vi "Sweep Mode (Read).vi"(6 "ISOBUS address":T5=-1 caption="ISOBUS address (-1)", 8 "error in":errorcluster, 11 "Mercury Reference In":T2) -> (0 "error out":errorcluster, 2 "Sweep Mode":string, 3 "Mercury Reference Out":T2, 4 "Valid?":T1)   [LabVIEW 2013, in "Mercury iXX.lvlib" / "Control Loop.lvlib"]
doc: "Check the sweep mode of the control loop."
uses:
  <instrlib>/Mercury iXX/Public/Libraries/Control Loop.lvlib
  <instrlib>/Mercury iXX/Public/Controls/Mercury Reference.ctl
  <instrlib>/Mercury iXX/Public/Controls/Comms Transport Layer.ctl
  <instrlib>/Mercury iXX/Private/Controls/Query Dynamic Reference.ctl
  <instrlib>/Mercury iXX/Public/Controls/ISOBus Address.ctl
  <instrlib>/Mercury iXX/Public/Controls/Is Valid LED.ctl
  <instrlib>/Mercury iXX/Private/Controls/Command Verbs.ctl
  <instrlib>/Mercury iXX/Mercury iXX.lvlib
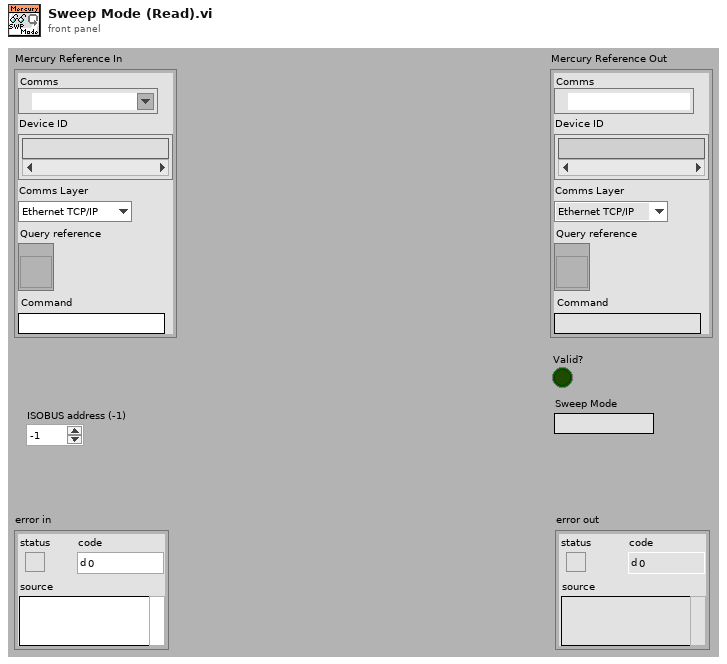
[diagram p1: front panel]
types:
  T1 = typedef "Mercury iXX.lvlib/Is Valid LED.ctl" = bool
  T2 = typedef "Mercury iXX.lvlib/Mercury Reference.ctl" = cluster{"Comms":refnum<visa-resource-name>, "Device ID":string[], "Comms Layer":T3, "Command":string, "Query reference":T4}
  T3 = typedef "Mercury iXX.lvlib/Comms Transport Layer.ctl" = enum16{"Ethernet TCP/IP", "USB", "ISOBus - RS-232", "GPIB"}
  T4 = typedef "Mercury iXX.lvlib/Query Dynamic Reference.ctl" = refnum<vi>
  T5 = typedef "Mercury iXX.lvlib/ISOBus Address.ctl" = i32
  T6 = typedef "Mercury iXX.lvlib/Command Verbs.ctl" = string
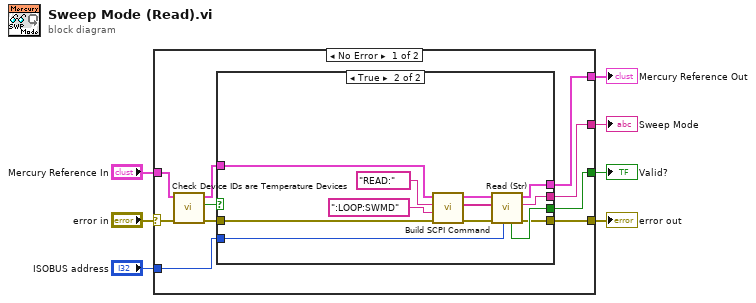
[diagram p0: block diagram]
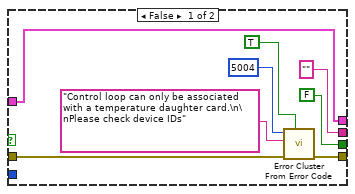
[diagram p2: hidden frame]
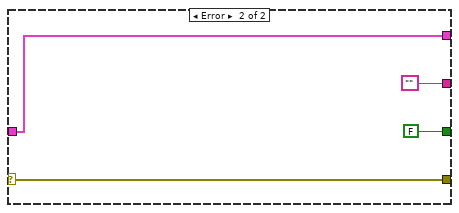
[diagram p3: hidden frame]
diagram:
  n1 = case shown="No Error" "error in" {
    selector: "error in" -> [w13 w40]
    tunnel: "Mercury Reference In" -> [w11 w41]
    tunnel: [w17 w41] -> w4
    tunnel: [w15 w40] -> w5
    tunnel: "ISOBUS address" -> [w16 _]
    tunnel: [w8 ""] -> w1
    tunnel: [w9 FALSE ("Valid?")] -> w2
    frame No Error {
      n2 = call <instrlib>:"Check Device IDs are Temperature Devices.vi"("error in"=w13, "Mercury Reference In"=w11) -> ("error out"=w12:errorcluster, "Valid?"=w14:bool, "Mercury Reference Out"=w10:T2)  [unwired: 7 out]
      n3 = case shown="True" w14 {
        tunnel: w10 -> [w25 w32]
        tunnel: [w25 w27] -> w17
        tunnel: w12 -> [w23 w31]
        tunnel: w16 -> [_ w30]
        tunnel: [w24 w26] -> w15
        tunnel: [T1 FALSE ("Valid?") w29] -> w9
        tunnel: ["" ("Response") w28] -> w8
        frame False {
          n4 = call <vilib>:"Error Cluster From Error Code.vi"("show call chain? (False)"=TRUE, "error in (no error)"=w23, "error message (\"\")"="Control loop can only be associated with a temperature daughter card.\n\nPlease check device IDs" ("error message (\"\")"), "error code (0)"=5004) -> ("error out"=w24:errorcluster)  [unwired: 5 out]
        }
        frame True {
          n5 = call <instrlib>:"Build SCPI Command.vi"("error in"=w31, "Noun(s)"=":LOOP:SWMD" ("Command"), "Verb"=T6 "READ:", "Mercury Reference In"=w32) -> ("error out"=w33:errorcluster, "SCPI Message(s)"=w36:string[], "Mercury Reference Out"=w35:T2)  [unwired: 5 out]
          n6 = call <instrlib>:"Read (Str).vi"("ISOBUS address"=w30, "error in"=w33, "SCPI Message(s)"=w36, "Mercury Reference In"=w35) -> ("error out"=w26:errorcluster, "Response"=w28:string, "Mercury Reference Out"=w27:T2, "Valid?"=w29:T1)  [unwired: 4 out]
        }
      }
    }
    frame Error {
    }
  }
  "Mercury Reference Out" <- w4
  "Sweep Mode" <- w1
  "error out" <- w5
  "Valid?" <- w2
